vi "remotecontrol.vi"() -> ()   [LabVIEW 2013]
panel:
  in  "standar function cluster":T1={"Duty Cycle (50.0)"=50.0, "waveform"=0, "Pulse Delay"=0.0, "amplitude (1)"=1.0} {"waveform" items=["Square"=2, "Pulse"=1002, "Ramp"=1001, "Noise"=1003, "DC"=6, "sin(x)/x"=1004, "Gaussian"=1005, "Lorentz"=1006, "Exponential Decay"=1008, "Exponential Rise"=1007, "Sine"=1, "Haversine"=1009]}
  in  "channel control cluster":T2 {"reference clock source (0: Internal)" items=["Internal", "External"]; "operation mode" items=["Modulation"=1001, "Continous"=0, "Burst"=1, "Sweep"=1002]; "outpout mode" items=["Standard Waveform", "Arbitrary Waveform"]}
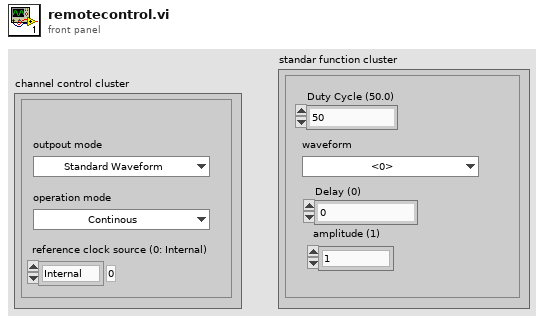
[diagram p1: front panel]
types:
  T1 = cluster{"Duty Cycle (50.0)":dbl, "waveform":i32, "Pulse Delay":dbl, "amplitude (1)":dbl}
  T2 = cluster{"outpout mode":i32, "operation mode":i32, "reference clock source (0: Internal)":i32}
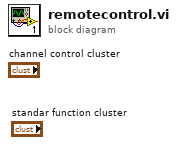
[diagram p0: block diagram]
diagram:
